vi "program 4.vi"() -> ()   [LabVIEW 2020]
panel:
  in  "Pokaz w. krytyczne":bool
  out "XY Graph":cluster{dbl[], dbl[]}[](graph)
  in  "stop":bool
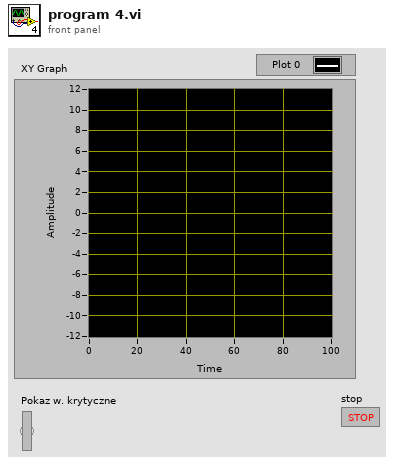
[diagram p1: front panel]
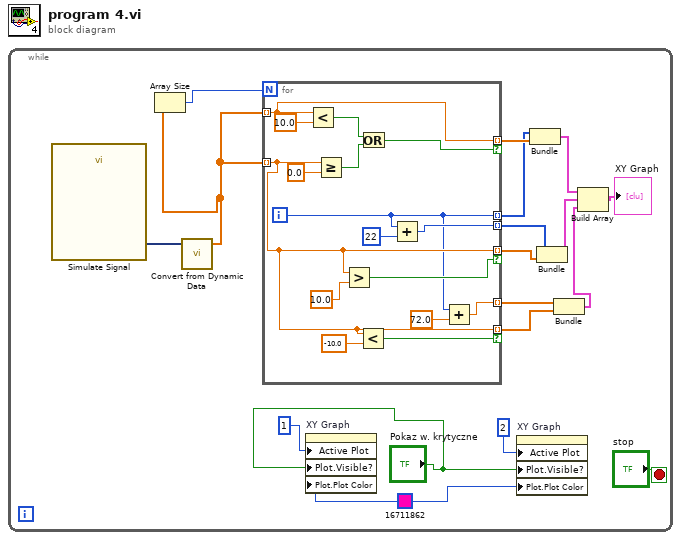
[diagram p0: block diagram]
diagram:
  n1 = while {
    stop <- "stop" stop-if-true
    w3 = u32 16711862 ("Plot.Plot Color")
    n2 = call "Simulate Signal"() -> ("Sine with Uniform Noise"=w17:dynamicdata)  [unwired: 14 in, 1 out]
    n3 = call "Convert from Dynamic Data"("Dynamic Data Type"=w17) -> ("Array"=w14:dbl[])  [unwired: 3 in]
    n4 = Array Size(array=w14) -> (size(s)=w13:i32)
    n5 = for {
      N: w13 -> [_]
      tunnel: w14 -> [w29] mode=indexing
      tunnel: w14 -> [w23] mode=indexing
      tunnel: [w29] -> w16 mode=indexing if=w30
      tunnel: [w20] -> w15 mode=indexing
      tunnel: [w23] -> w10 mode=indexing if=w27
      tunnel: [w26] -> w9 mode=indexing
      tunnel: [w23] -> w6 mode=indexing if=w22
      tunnel: [w19] -> w5 mode=indexing
      i -> [w20]
      n6 = Less?(x=w29, y=10.0) -> (x < y?=w31:bool)
      n7 = Greater Or Equal?(x=w23, y=0.0) -> (x >= y?=w32:bool)
      n8 = Greater?(x=w23, y=10.0) -> (0:w27:bool)
      n9 = Less?(x=w23, y=-10.0) -> (x < y?=w22:bool)
      n10 = Or(x=w31, y=w32) -> (x .or. y?=w30:bool)
      n11 = Add(x=w20, y=22) -> (x+y=w26:i32)
      n12 = Add(x=w20, y=72.0) -> (x+y=w19:dbl)
    }
    n13 = property on="XY Graph" class="XYGraph (strict)"("Active Plot"=u32 1, "Plot.Visible?"="Pokaz w. krytyczne", "Plot.Plot Color"=w3) -> ()  [unwired: 2 in, 2 out]
    n14 = property on="XY Graph" class="XYGraph (strict)"("Active Plot"=u32 2, "Plot.Visible?"="Pokaz w. krytyczne", "Plot.Plot Color"=w3) -> ()  [unwired: 2 in, 2 out]
    n15 = Bundle(w15, w16) -> (w12:cluster{i32[], dbl[]})  [unwired: 1 in]
    n16 = Bundle(w9, w10) -> (w8:cluster{i32[], dbl[]})  [unwired: 1 in]
    n17 = Bundle(w5, w6) -> (w4:cluster{dbl[], dbl[]})  [unwired: 1 in]
    n18 = Build Array(w12, w8, w4) -> (→"XY Graph":cluster{dbl[], dbl[]}[])
  }
